vi "Multiple Connections - Server - TCP.vi"() -> ()   [LabVIEW 2011]
doc: "Demonstrates how to establish multiple connections and place them in a queue to be serviced. As connections are made, it sends the current date and time via TCP to all Client VIs that connect to it.\n\nThis VI has two parts -- a loop that listens for each client to connect, and a loop that sends the date and time to each connection in the queue.\n\n<B>Note:</B> Use this VI with Multiple Connections - Client 1.vi and Multiple Connections - Client 2.vi."
panel:
  out "# 2":i32
  in  "Port 2":u16=6342
  in  "stop":bool=TRUE
  out "# of Connections":i32
  in  "Port":u16=6341
  # "Instructions:\n1. Open the Multiple Connections - Client 1 and Client 2 VIs.\n2. Run this VI first.\n3. Run the Client VIs second and follow the instructions on their front panels.\n4. Stop This VI.  The Client VIs will stop on their own when they time out."
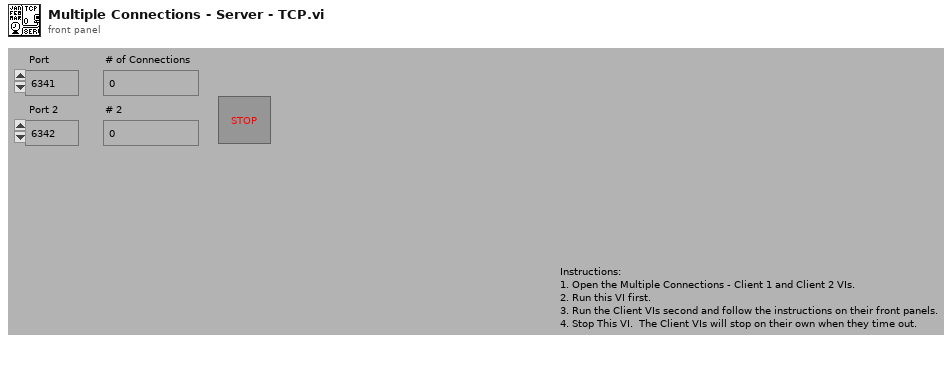
[diagram p1: front panel]
types:
  T1 = enum16{"Obtain", "Enqueue", "Dequeue", "Release"}
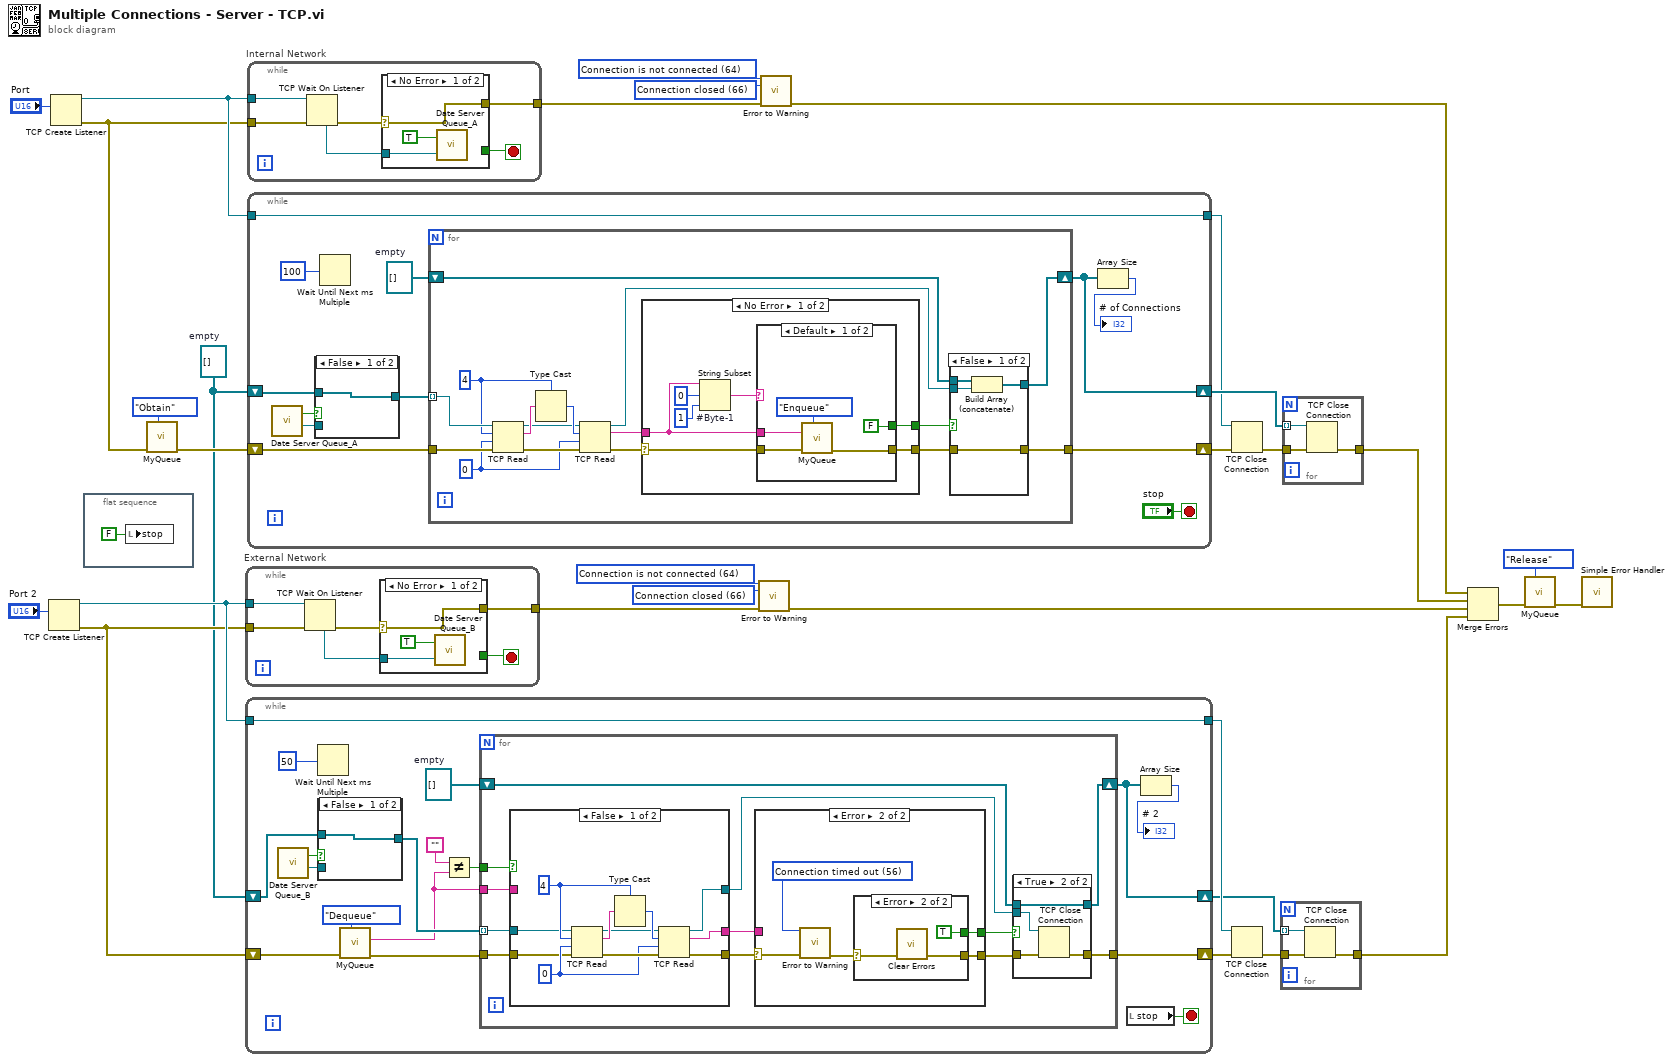
[diagram p0: block diagram]
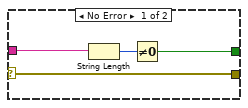
[diagram p2: hidden frame]
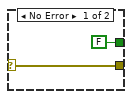
[diagram p3: hidden frame]
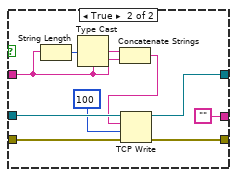
[diagram p4: hidden frame]
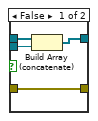
[diagram p5: hidden frame]
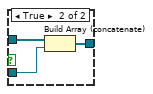
[diagram p6: hidden frame]
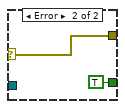
[diagram p7: hidden frame]
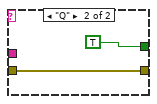
[diagram p8: hidden frame]
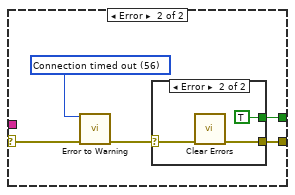
[diagram p9: hidden frame]
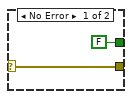
[diagram p10: hidden frame]
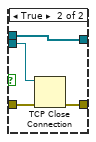
[diagram p11: hidden frame]
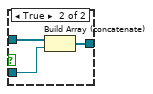
[diagram p12: hidden frame]
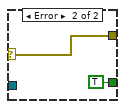
[diagram p13: hidden frame]
diagram:
  w13 = 66 items=["No Error", "Argument Error", "Memory Full", "Out of Zone", "End of File", "File Already Open", "Generic File IO Error", "File Not Found", "File Permission Error", "Disk Full", "Duplicate Path", "Too Many Files Open", "Not Enabled", "Resource File Not Found", "Cannot Add Resource", "Resource Not Found", "Image Not Found", "Image Memory Error", "Pen Does Not Exist", "Config Bad Type", "Config Token Not Found", "Config Parse Error", "Config Memory Error", "Bad External Code Format", "Bad External Code Offset", "External Code Not Present", "Null Window", "Destroy Window Mixup", "Null Menu", "Print Aborted", "Bad Print Record", "Print Driver Error", "Windows Error During Print", "Memory Error During Print", "Print Dialog Error", "Generic Print Error", "Invalid Device Refnum", "Device Not Found", "Device Parameter Error", "Device Unit Error", "Can't Open Device", "Device Call Aborted", "Generic Error", "Cancelled By User", "Object ID Too Low", "Object ID Too High", "Object Not In Heap", "Unknown Heap", "Bad DefProc ID", "DefProc Not In Table", "Message Out Of Range", "Null Method", "Unknown Message", "Manager Call Not Supported", "Bad address", "Connection In progress", "Connection timed out", "Connection is already in progress", "Network attribute not supported", "Network error", "Address in use", "System out of memory", "Connection aborted", "Connection refused", "Connection is not connected", "Connection is already connected", "Connection closed", "Initialize error (interapplication manager)", "Bad occurrence", "Wait on unbound occurrence handler", "Occurrence queue overflow", "Bad path", "Semaphore not signaled", "Unrecognized type (interapplication manager)"] ("2nd Error to Convert")
  w12 = 64 items=["No Error", "Argument Error", "Memory Full", "Out of Zone", "End of File", "File Already Open", "Generic File IO Error", "File Not Found", "File Permission Error", "Disk Full", "Duplicate Path", "Too Many Files Open", "Not Enabled", "Resource File Not Found", "Cannot Add Resource", "Resource Not Found", "Image Not Found", "Image Memory Error", "Pen Does Not Exist", "Config Bad Type", "Config Token Not Found", "Config Parse Error", "Config Memory Error", "Bad External Code Format", "Bad External Code Offset", "External Code Not Present", "Null Window", "Destroy Window Mixup", "Null Menu", "Print Aborted", "Bad Print Record", "Print Driver Error", "Windows Error During Print", "Memory Error During Print", "Print Dialog Error", "Generic Print Error", "Invalid Device Refnum", "Device Not Found", "Device Parameter Error", "Device Unit Error", "Can't Open Device", "Device Call Aborted", "Generic Error", "Cancelled By User", "Object ID Too Low", "Object ID Too High", "Object Not In Heap", "Unknown Heap", "Bad DefProc ID", "DefProc Not In Table", "Message Out Of Range", "Null Method", "Unknown Message", "Manager Call Not Supported", "Bad address", "Connection In progress", "Connection timed out", "Connection is already in progress", "Network attribute not supported", "Network error", "Address in use", "System out of memory", "Connection aborted", "Connection refused", "Connection is not connected", "Connection is already connected", "Connection closed", "Initialize error (interapplication manager)", "Bad occurrence", "Wait on unbound occurrence handler", "Occurrence queue overflow", "Bad path", "Semaphore not signaled", "Unrecognized type (interapplication manager)"] ("1st Error to Convert")
  w4 = refnum<k5>[] []  # empty
  w25 = 66 items=["No Error", "Argument Error", "Memory Full", "Out of Zone", "End of File", "File Already Open", "Generic File IO Error", "File Not Found", "File Permission Error", "Disk Full", "Duplicate Path", "Too Many Files Open", "Not Enabled", "Resource File Not Found", "Cannot Add Resource", "Resource Not Found", "Image Not Found", "Image Memory Error", "Pen Does Not Exist", "Config Bad Type", "Config Token Not Found", "Config Parse Error", "Config Memory Error", "Bad External Code Format", "Bad External Code Offset", "External Code Not Present", "Null Window", "Destroy Window Mixup", "Null Menu", "Print Aborted", "Bad Print Record", "Print Driver Error", "Windows Error During Print", "Memory Error During Print", "Print Dialog Error", "Generic Print Error", "Invalid Device Refnum", "Device Not Found", "Device Parameter Error", "Device Unit Error", "Can't Open Device", "Device Call Aborted", "Generic Error", "Cancelled By User", "Object ID Too Low", "Object ID Too High", "Object Not In Heap", "Unknown Heap", "Bad DefProc ID", "DefProc Not In Table", "Message Out Of Range", "Null Method", "Unknown Message", "Manager Call Not Supported", "Bad address", "Connection In progress", "Connection timed out", "Connection is already in progress", "Network attribute not supported", "Network error", "Address in use", "System out of memory", "Connection aborted", "Connection refused", "Connection is not connected", "Connection is already connected", "Connection closed", "Initialize error (interapplication manager)", "Bad occurrence", "Wait on unbound occurrence handler", "Occurrence queue overflow", "Bad path", "Semaphore not signaled", "Unrecognized type (interapplication manager)"] ("2nd Error to Convert")
  w26 = 64 items=["No Error", "Argument Error", "Memory Full", "Out of Zone", "End of File", "File Already Open", "Generic File IO Error", "File Not Found", "File Permission Error", "Disk Full", "Duplicate Path", "Too Many Files Open", "Not Enabled", "Resource File Not Found", "Cannot Add Resource", "Resource Not Found", "Image Not Found", "Image Memory Error", "Pen Does Not Exist", "Config Bad Type", "Config Token Not Found", "Config Parse Error", "Config Memory Error", "Bad External Code Format", "Bad External Code Offset", "External Code Not Present", "Null Window", "Destroy Window Mixup", "Null Menu", "Print Aborted", "Bad Print Record", "Print Driver Error", "Windows Error During Print", "Memory Error During Print", "Print Dialog Error", "Generic Print Error", "Invalid Device Refnum", "Device Not Found", "Device Parameter Error", "Device Unit Error", "Can't Open Device", "Device Call Aborted", "Generic Error", "Cancelled By User", "Object ID Too Low", "Object ID Too High", "Object Not In Heap", "Unknown Heap", "Bad DefProc ID", "DefProc Not In Table", "Message Out Of Range", "Null Method", "Unknown Message", "Manager Call Not Supported", "Bad address", "Connection In progress", "Connection timed out", "Connection is already in progress", "Network attribute not supported", "Network error", "Address in use", "System out of memory", "Connection aborted", "Connection refused", "Connection is not connected", "Connection is already connected", "Connection closed", "Initialize error (interapplication manager)", "Bad occurrence", "Wait on unbound occurrence handler", "Occurrence queue overflow", "Bad path", "Semaphore not signaled", "Unrecognized type (interapplication manager)"] ("1st Error to Convert")
  n1 = TCP Create Listener(10:"Port 2") -> (0:w5:errorcluster, 3:w10:refnum<k5>)  [unwired: 1 in, 4 out]
  n2 = TCP Create Listener(10:"Port") -> (0:w19:errorcluster, 3:w28:refnum<k5>)  [unwired: 1 in, 4 out]
  n3 = flat-sequence {
    frame #0 {
      n4 = local write "stop"(FALSE ("stop")) -> ()
    }
  }
  n5 = call "MyQueue.vi"("Mode"=T1."Obtain", "error in (no error)"=w19) -> ("error out"=w21:errorcluster)  [unwired: 8 in, 1 out]
  n6 = while "External Network" {
    tunnel: w10 -> [w36]
    tunnel: w5 -> [w37]
    tunnel: [w32] -> w11
    stop <- w33 stop-if-true
    n7 = TCP Wait On Listener(8:w37, 11:w36) -> (0:w34:errorcluster, 4:w35:refnum<k5>)  [unwired: 5 out]
    n8 = case shown="No Error" w34 {
      selector: w34 -> [w38 w41]
      tunnel: w35 -> [w39 _]
      tunnel: [_ TRUE] -> w33
      tunnel: [w38 w41] -> w32
      frame No Error {
        n9 = call "Date Server Queue_B.vi"("new value"=w39, "set queue? (F: de-queue)"=TRUE) -> ()  [unwired: 2 out]
      }
      frame Error {
      }
    }
  }
  n10 = while {
    shift-left: w4 -> [w57]
    shift-right: [w54] -> w8
    tunnel: w10 -> [w52]
    tunnel: [w52] -> w9
    shift-right: [w51] -> w16
    shift-left: w5 -> [w49]
    stop <- w47 stop-if-true
    w55 = refnum<k5>[] []  # empty
    n11 = call "Date Server Queue_B.vi"() -> ("value"=w59:refnum<k5>, "valid?"=w58:bool)  [unwired: 2 in]
    n12 = Wait Until Next ms Multiple(millisecond multiple=u32 50) -> ()  [unwired: 1 out]
    n13 = case shown="False" w58 {
      tunnel: w59 -> [_ w118]
      tunnel: w57 -> [w115 w117]
      tunnel: [w115 w116] -> w56
      frame False {
      }
      frame True {
        n14 = Build Array (concatenate)(w117, w118) -> (w116:refnum<k5>[])
      }
    }
    n15 = call "MyQueue.vi"("Mode"=T1."Dequeue", "error in (no error)"=w49) -> ("error out"=w48:errorcluster, "Queue Out"=w44:string)  [unwired: 8 in]
    n16 = Not Equal?(x="", y=w44) -> (x != y?=w43:bool)
    n17 = for {
      tunnel: w56 -> [w68] mode=indexing
      shift-right: [w69] -> w54
      shift-left: w55 -> [w71]
      tunnel: [w70] -> w51
      tunnel: w48 -> [w67]
      tunnel: w44 -> [w62]
      tunnel: w43 -> [w61]
      n18 = case shown="False" w61 {
        tunnel: w68 -> [w88 w102]
        tunnel: w67 -> [w90 w104]
        tunnel: [w89 w100] -> w66
        tunnel: w62 -> [_ w103]
        tunnel: [w86 w98] -> w60
        tunnel: [w87 ""] -> w63
        frame False {
          w91 = 0 ("timeout ms (25000)")
          w93 = 4
          n19 = TCP Read(connection ID=w88, bytes to read=w93, error in (no error)=w90, 9:w91) -> (connection ID out=w92:refnum<k5>, data out=w94:string, error out=w95:errorcluster)  [unwired: 1 out]
          n20 = Type Cast(type=w93, x=w94) -> (*(type *) &x=w96:i32)
          n21 = TCP Read(connection ID=w92, bytes to read=w96, error in (no error)=w95, 9:w91) -> (connection ID out=w86:refnum<k5>, data out=w87:string, error out=w89:errorcluster)  [unwired: 1 out]
        }
        frame True {
          n22 = String Length(string=w103) -> (length=w106:i32)
          n23 = Type Cast(type=w103, x=w106) -> (*(type *) &x=w105:string)
          n24 = Concatenate Strings(w105, w103) -> (w99:string)
          n25 = TCP Write(connection ID=w102, data in=w99, error in (no error)=w104, 9:100 ("timeout ms (25000)")) -> (connection ID out=w98:refnum<k5>, error out=w100:errorcluster)  [unwired: 1 out]
        }
      }
      n26 = case shown="Error" w66 {
        selector: w66 -> [w75 w80]
        tunnel: [w75 w77] -> w64
        tunnel: [w72 w76] -> w65
        tunnel: w63 -> [w74 _]
        frame No Error {
          n27 = String Length(string=w74) -> (length=w73:i32)
          n28 = Not Equal To 0?(x=w73) -> (x != 0?=w72:bool)
        }
        frame Error {
          w79 = 56 items=["No Error", "Argument Error", "Memory Full", "Out of Zone", "End of File", "File Already Open", "Generic File IO Error", "File Not Found", "File Permission Error", "Disk Full", "Duplicate Path", "Too Many Files Open", "Not Enabled", "Resource File Not Found", "Cannot Add Resource", "Resource Not Found", "Image Not Found", "Image Memory Error", "Pen Does Not Exist", "Config Bad Type", "Config Token Not Found", "Config Parse Error", "Config Memory Error", "Bad External Code Format", "Bad External Code Offset", "External Code Not Present", "Null Window", "Destroy Window Mixup", "Null Menu", "Print Aborted", "Bad Print Record", "Print Driver Error", "Windows Error During Print", "Memory Error During Print", "Print Dialog Error", "Generic Print Error", "Invalid Device Refnum", "Device Not Found", "Device Parameter Error", "Device Unit Error", "Can't Open Device", "Device Call Aborted", "Generic Error", "Cancelled By User", "Object ID Too Low", "Object ID Too High", "Object Not In Heap", "Unknown Heap", "Bad DefProc ID", "DefProc Not In Table", "Message Out Of Range", "Null Method", "Unknown Message", "Manager Call Not Supported", "Bad address", "Connection In progress", "Connection timed out", "Connection is already in progress", "Network attribute not supported", "Network error", "Address in use", "System out of memory", "Connection aborted", "Connection refused", "Connection is not connected", "Connection is already connected", "Connection closed", "Initialize error (interapplication manager)", "Bad occurrence", "Wait on unbound occurrence handler", "Occurrence queue overflow", "Bad path", "Semaphore not signaled", "Unrecognized type (interapplication manager)"] ("1st Error to Convert")
          n29 = call <vilib>:"Error to Warning.vi"("1st Error to Convert"=w79, "error in"=w80) -> ("warning out"=w78:errorcluster)  [unwired: 13 in]
          n30 = case shown="Error" w78 {
            selector: w78 -> [w82 w85]
            tunnel: [w82 w84] -> w77
            tunnel: [FALSE TRUE] -> w76
            frame No Error {
            }
            frame Error {
              n31 = call <vilib>:"Clear Errors.vi"("error in (no error)"=w85) -> ("error out"=w84:errorcluster)  [unwired: 6 in]
            }
          }
        }
      }
      n32 = case shown="True" w65 {
        tunnel: w71 -> [w110 w114]
        tunnel: w60 -> [w109 w113]
        tunnel: [w108 w114] -> w69
        tunnel: w64 -> [w107 w112]
        tunnel: [w107 w111] -> w70
        frame False {
          n33 = Build Array (concatenate)(w110, w109) -> (w108:refnum<k5>[])
        }
        frame True {
          n34 = TCP Close Connection(connection ID=w113, error in (no error)=w112) -> (error out=w111:errorcluster)  [unwired: 2 out]
        }
      }
    }
    n35 = local read "stop"() -> (w47:bool)
    n36 = Array Size(array=w54) -> (size(s)=→"# 2":i32)
  }
  n37 = while "Internal Network" {
    tunnel: w28 -> [w123]
    tunnel: w19 -> [w124]
    tunnel: [w119] -> w27
    stop <- w120 stop-if-true
    n38 = TCP Wait On Listener(8:w124, 11:w123) -> (0:w121:errorcluster, 4:w122:refnum<k5>)  [unwired: 5 out]
    n39 = case shown="No Error" w121 {
      selector: w121 -> [w125 w128]
      tunnel: w122 -> [w126 _]
      tunnel: [_ TRUE] -> w120
      tunnel: [w125 w128] -> w119
      frame No Error {
        n40 = call "Date Server Queue_A.vi"("new value"=w126, "set queue? (F: de-queue)"=TRUE) -> ()  [unwired: 2 out]
      }
      frame Error {
      }
    }
  }
  n41 = while {
    shift-left: w4 -> [w139]
    shift-right: [w136] -> w30
    tunnel: w28 -> [w134]
    tunnel: [w134] -> w29
    shift-right: [w131] -> w20
    shift-left: w21 -> [w132]
    stop <- "stop" stop-if-true
    w137 = refnum<k5>[] []  # empty
    n42 = call "Date Server Queue_A.vi"() -> ("value"=w141:refnum<k5>, "valid?"=w140:bool)  [unwired: 2 in]
    n43 = case shown="False" w140 {
      tunnel: w141 -> [_ w193]
      tunnel: w139 -> [w190 w192]
      tunnel: [w190 w191] -> w138
      frame False {
      }
      frame True {
        n44 = Build Array (concatenate)(w192, w193) -> (w191:refnum<k5>[])
      }
    }
    n45 = Wait Until Next ms Multiple(millisecond multiple=u32 100) -> ()  [unwired: 1 out]
    n46 = for {
      tunnel: w138 -> [w154] mode=indexing
      shift-right: [w156] -> w136
      shift-left: w137 -> [w157]
      tunnel: [w155] -> w131
      tunnel: w132 -> [w153]
      w142 = 0 ("timeout ms (25000)")
      w146 = 4
      n47 = TCP Read(connection ID=w154, bytes to read=w146, error in (no error)=w153, 9:w142) -> (connection ID out=w145:refnum<k5>, data out=w147:string, error out=w149:errorcluster)  [unwired: 1 out]
      n48 = Type Cast(type=w146, x=w147) -> (*(type *) &x=w150:i32)
      n49 = TCP Read(connection ID=w145, bytes to read=w150, error in (no error)=w149, 9:w142) -> (connection ID out=w143:refnum<k5>, data out=w144:string, error out=w148:errorcluster)  [unwired: 1 out]
      n50 = case shown="No Error" w148 {
        selector: w148 -> [w158 w175]
        tunnel: [w161 w174] -> w152
        tunnel: [w160 w172] -> w151
        tunnel: w144 -> [w159 _]
        frame No Error {
          n51 = String Subset "#Byte-1"(string=w159, offset (0)=0, length (rest)=1 ("length (rest)")) -> (substring=w162:string)
          n52 = case shown="Default" w162 {
            tunnel: w159 -> [w165 _]
            tunnel: w158 -> [w167 w171]
            tunnel: [w166 w171] -> w161
            tunnel: [FALSE TRUE] -> w160
            frame Default {
              n53 = call "MyQueue.vi"("Mode"=T1."Enqueue", "error in (no error)"=w167, "Queue In"=w165) -> ("error out"=w166:errorcluster)  [unwired: 7 in, 1 out]
            }
            frame "Q" {
            }
          }
        }
        frame Error {
          w176 = 56 items=["No Error", "Argument Error", "Memory Full", "Out of Zone", "End of File", "File Already Open", "Generic File IO Error", "File Not Found", "File Permission Error", "Disk Full", "Duplicate Path", "Too Many Files Open", "Not Enabled", "Resource File Not Found", "Cannot Add Resource", "Resource Not Found", "Image Not Found", "Image Memory Error", "Pen Does Not Exist", "Config Bad Type", "Config Token Not Found", "Config Parse Error", "Config Memory Error", "Bad External Code Format", "Bad External Code Offset", "External Code Not Present", "Null Window", "Destroy Window Mixup", "Null Menu", "Print Aborted", "Bad Print Record", "Print Driver Error", "Windows Error During Print", "Memory Error During Print", "Print Dialog Error", "Generic Print Error", "Invalid Device Refnum", "Device Not Found", "Device Parameter Error", "Device Unit Error", "Can't Open Device", "Device Call Aborted", "Generic Error", "Cancelled By User", "Object ID Too Low", "Object ID Too High", "Object Not In Heap", "Unknown Heap", "Bad DefProc ID", "DefProc Not In Table", "Message Out Of Range", "Null Method", "Unknown Message", "Manager Call Not Supported", "Bad address", "Connection In progress", "Connection timed out", "Connection is already in progress", "Network attribute not supported", "Network error", "Address in use", "System out of memory", "Connection aborted", "Connection refused", "Connection is not connected", "Connection is already connected", "Connection closed", "Initialize error (interapplication manager)", "Bad occurrence", "Wait on unbound occurrence handler", "Occurrence queue overflow", "Bad path", "Semaphore not signaled", "Unrecognized type (interapplication manager)"] ("1st Error to Convert")
          n54 = call <vilib>:"Error to Warning.vi"("1st Error to Convert"=w176, "error in"=w175) -> ("warning out"=w173:errorcluster)  [unwired: 13 in]
          n55 = case shown="Error" w173 {
            selector: w173 -> [w178 w181]
            tunnel: [w178 w180] -> w174
            tunnel: [FALSE TRUE] -> w172
            frame No Error {
            }
            frame Error {
              n56 = call <vilib>:"Clear Errors.vi"("error in (no error)"=w181) -> ("error out"=w180:errorcluster)  [unwired: 6 in]
            }
          }
        }
      }
      n57 = case shown="False" w151 {
        tunnel: w157 -> [w185 w189]
        tunnel: w143 -> [w184 w188]
        tunnel: [w183 w189] -> w156
        tunnel: w152 -> [w182 w187]
        tunnel: [w182 w186] -> w155
        frame False {
          n58 = Build Array (concatenate)(w185, w184) -> (w183:refnum<k5>[])
        }
        frame True {
          n59 = TCP Close Connection(connection ID=w188, error in (no error)=w187) -> (error out=w186:errorcluster)  [unwired: 2 out]
        }
      }
    }
    n60 = Array Size(array=w136) -> (size(s)=→"# of Connections":i32)
  }
  n61 = call <vilib>:"Error to Warning.vi"("1st Error to Convert"=w12, "2nd Error to Convert"=w13, "error in"=w11) -> ("warning out"=w7:errorcluster)  [unwired: 2 in, 10 out]
  n62 = call <vilib>:"Error to Warning.vi"("1st Error to Convert"=w26, "2nd Error to Convert"=w25, "error in"=w27) -> ("warning out"=w22:errorcluster)  [unwired: 2 in, 10 out]
  n63 = TCP Close Connection(connection ID=w29, error in (no error)=w20) -> (error out=w23:errorcluster)  [unwired: 2 out]
  n64 = TCP Close Connection(connection ID=w9, error in (no error)=w16) -> (error out=w15:errorcluster)  [unwired: 2 out]
  n65 = for {
    tunnel: w8 -> [w196] mode=indexing
    tunnel: [w195] -> w6
    tunnel: w15 -> [w194]
    n66 = TCP Close Connection(connection ID=w196, error in (no error)=w194) -> (error out=w195:errorcluster)  [unwired: 2 out]
  }
  n67 = for {
    tunnel: w30 -> [w199] mode=indexing
    tunnel: [w198] -> w3
    tunnel: w23 -> [w197]
    n68 = TCP Close Connection(connection ID=w199, error in (no error)=w197) -> (error out=w198:errorcluster)  [unwired: 2 out]
  }
  n69 = Merge Errors(w22, w3, w7, w6) -> (w2:errorcluster)
  n70 = call "MyQueue.vi"("Mode"=T1."Release", "error in (no error)"=w2) -> ("error out"=w1:errorcluster)  [unwired: 8 in, 1 out]
  n71 = call <vilib>:"Simple Error Handler.vi"("error in (no error)"=w1) -> ()  [unwired: 1 in, 8 out]
